vi "ROI entry-Event handler-Completion.vi"(11 "Ctrl ref of the control that caused the user event":refnum<vi>) -> (1 "Exit":bool=TRUE, 3 "Imaging Mode":T1)   [LabVIEW 2013]
uses:
  Typedefs/Top level VI states.ctl
  Visualisation/Functional Imaging Viewer/SubVIs/Experiment header interface/Typedefs/Header file type enum.ctl
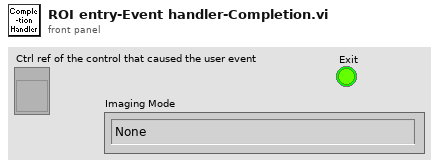
[diagram p1: front panel]
types:
  T1 = typedef "Top level VI states.ctl" = enum16{"None", "Initialise UI", "<STACK PROTOCOL STATES>", "AOL Zstack-START", "AOL Zstack-STOP", "Motor Zstack-START", "Motor Zstack-STOP", "<ACQUISITION PROTOCOL STATES> ", "Functional Acquisition-START", "Functional Acquisition-STOP", "Single Plane Acquisition-START", "Single Plane Acquisition-STOP", "Volume Acquisition-START", "Volume Acquisition-STOP", "<LIVE IMAGING PROTOCOL STATES>", "Live Imaging-START", "Live Imaging-STOP", "Live Plane Imaging-START", "Live Plane Imaging-STOP", "Live Volume Imaging-START", "Live Volume Imaging-STOP", "EXIT"}
  T2 = typedef "Header file type enum.ctl" = enum16{"All parameters", "Params for funct acq w ROI or mscn", "Params for funct acq w rectangles", "Live imaging header parameters", "AOL Parameters"}
  T3 = typedef "ROI parameters data type.ctl" = cluster{"ROI index":dbl, "ROI ID":dbl, "ROI Time (ns)":dbl, "Pixels in ROI":dbl, "X start":dbl, "Y start":dbl, "Z start":dbl, "X stop":dbl, "Y stop":dbl, "Z stop":dbl, "Angle (deg)":dbl, "Composite ID":dbl, "Number of lines":dbl, "Frame Size":dbl, "Zoom":dbl, "Laser Power (%)":dbl, "ROI group ID":dbl}
  T4 = typedef "AOL_Globals.ctl" = cluster{"Imaging Protocol":T5, "Number of POI":u16, "Number of Miniscans":u16, "Number of Trials":u16, "Number of Cycles ":u64, "# Averaged Frames":u16, "Laser power (%)":u8, "Pockels":dbl, "Acquisition Length (sec)":dbl, "Fill time (us)":dbl, "POI Dwell time (us)":dbl, "Miniscan Dwell time per pixel (us)":dbl, "PMT 1":dbl, "PMT 2":dbl, "Back Apperture":dbl, "Frame Size":T6, "Center Frequency":dbl, "Field of View":dbl, "DwellTime (us)":dbl, "Wavelength (nm)":dbl, "Zoom":dbl, "AOL Z":dbl, "AOL Mode":T7, "GridXY":dbl, "GridZ":dbl, "TriggerPeriod (sec)":dbl, "Number of Pixels in Miniscan":u16, "Experiment folder path":path, "X centre":dbl, "Y centre":dbl, "Angle (degrees)":dbl, "Plane Mode":T8, "Threshold":u16[], "Regenerate Chirps":bool, "Rectangle ROI length (pixels)":u16, "Rectangle ROI height (pixels)":u16, "AOD fill":u16, "Samples Wait after Trigger":u16, "StartUp Delay":i32, "Slip Cycle":u32, "Add Cycle":bool}
  T5 = typedef "Imaging Protocols enum.ctl" = enum16{"AOL Z-Stack", "Motor Z Stack", "Functional Acquisition", "Single Plane Acquisition", "Volume Acquisition", "Live Imaging", "Live Plane Imaging", "Live Volume Imaging"}
  T6 = typedef "Frame Size.ctl" = u16
  T7 = typedef "AOL modes.ctl" = enum16{"Raster", "Structural", "Pointing", "Mini Scan", "Alignment"}
  T8 = typedef "Plane Mode.ctl" = u16
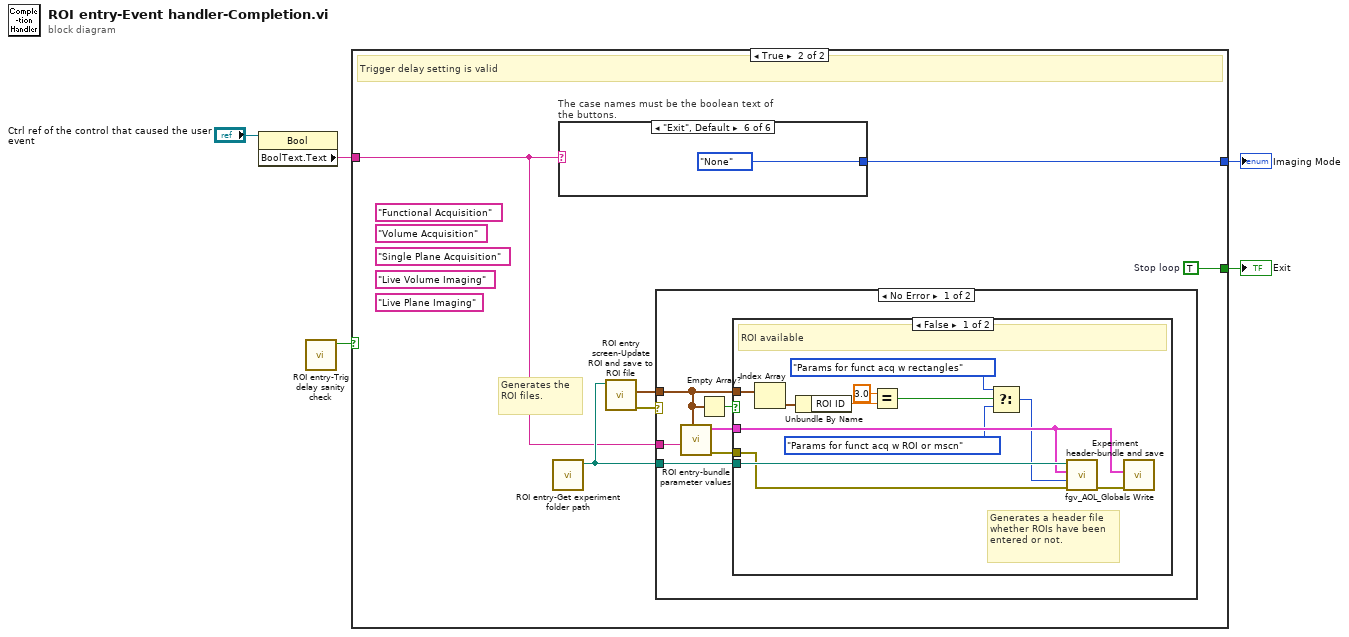
[diagram p0: block diagram]
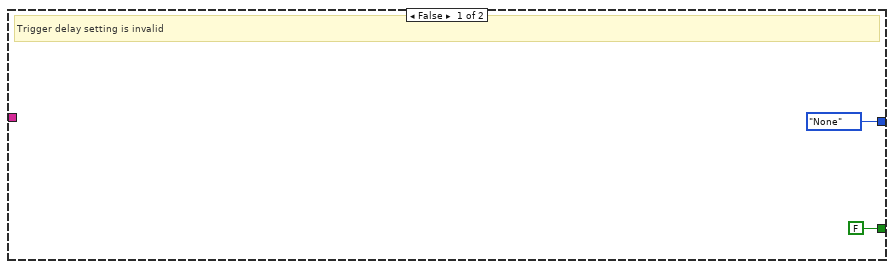
[diagram p2: hidden frame]
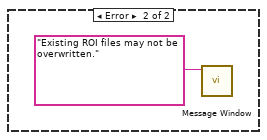
[diagram p4: hidden frame]
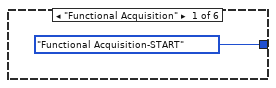
[diagram p5: hidden frame]
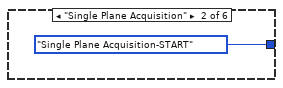
[diagram p6: hidden frame]
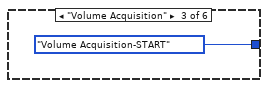
[diagram p7: hidden frame]
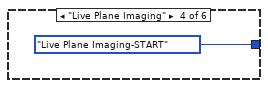
[diagram p8: hidden frame]
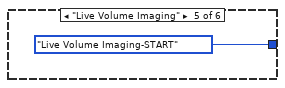
[diagram p9: hidden frame]
diagram:
  n1 = property on="Property Node" class="Bool"(reference="Ctrl ref of the control that caused the user event") -> ("BoolText.Text"=w5:string)  [unwired: 1 in, 2 out]
  n2 = call "ROI entry-Trig delay sanity check.vi"() -> ("Trigger delay is valid"=w1:bool)  [unwired: 10 in, 1 out]
  n3 = case shown="True" w1 {
    tunnel: w5 -> [_ w12]
    tunnel: [Top_level_VI_states."None" ("Imaging Mode") w9] -> w4
    tunnel: [FALSE ("Stop loop") w8] -> w2
    frame False {
      # "Trigger delay setting is invalid"
    }
    frame True {
      w8 = TRUE  # Stop loop
      (unwired) "Live Plane Imaging" ("Boolean Text.Text")
      (unwired) "Single Plane Acquisition" ("Boolean Text.Text")
      (unwired) "Live Volume Imaging" ("Boolean Text.Text")
      (unwired) "Functional Acquisition" ("Boolean Text.Text")
      (unwired) "Volume Acquisition" ("Boolean Text.Text")
      # "Generates the ROI files."
      # "Trigger delay setting is valid"
      n4 = call "ROI entry-Get experiment folder path.vi"() -> ("Experiment folder path"=w13:path)  [unwired: 10 in, 1 out]
      n5 = case "The case names must be the boolean text of the buttons." shown="\"Exit\", Default" w12 {
        tunnel: [Top_level_VI_states."Functional Acquisition-START" ("Imaging Mode") Top_level_VI_states."Single Plane Acquisition-START" ("Imaging Mode") Top_level_VI_states."Volume Acquisition-START" ("Imaging Mode") Top_level_VI_states."Live Plane Imaging-START" ("Imaging Mode") Top_level_VI_states."Live Volume Imaging-START" ("Imaging Mode") Top_level_VI_states."None" ("Imaging Mode")] -> w9
        frame "Functional Acquisition" {
        }
        frame "Single Plane Acquisition" {
        }
        frame "Volume Acquisition" {
        }
        frame "Live Plane Imaging" {
        }
        frame "Live Volume Imaging" {
        }
        frame "Exit", Default {
        }
      }
      n6 = call "ROI entry screen-Update ROI and save to ROI file.vi"("Experiment folder path"=w13) -> ("Error Out"=w11:errorcluster, "XYZ_Coordinates"=w10:T3[])  [unwired: 9 in]
      n7 = case shown="No Error" w11 {
        tunnel: w10 -> [w14 _]
        tunnel: w13 -> [w19 _]
        tunnel: w12 -> [w15 _]
        frame No Error {
          n8 = call "ROI entry-bundle parameter values.vi"("XYZ_Coordinates"=w14, "Button Label.Text"=w15) -> ("error out"=w17:errorcluster, "AOL_Globals out"=w18:T4)  [unwired: 8 in]
          n9 = Empty Array?(array=w14) -> (empty?=w16:bool)
          n10 = case shown="False" w16 {
            tunnel: w19 -> [w31 _]
            tunnel: w18 -> [w29 _]
            tunnel: w17 -> [w20 _]
            tunnel: w14 -> [w28 _]
            frame False {
              # "Generates a header file whether ROIs have been entered or not."
              # "ROI available"
              n11 = Index Array(array=w28) -> (element=w27:T3)  [unwired: 1 in]
              n12 = Unbundle By Name(w27) -> ("ROI ID"=w26:dbl)
              n13 = Equal?(x=3.0 ("y"), y=w26) -> (x = y?=w24:bool)
              n14 = Select(t=Header_file_type_enum."Params for funct acq w rectangles" ("Header file type"), s=w24, f=Header_file_type_enum."Params for funct acq w ROI or mscn" ("Header file type")) -> (s? t:f=w21:T2)
              n15 = call "Experiment header-bundle and save.vi"("error in (no error)"=w20, "Header file type"=w21, "AOL_Globals"=w29, "Experiment data folder path"=w31) -> ("error out"=w30:errorcluster)  [unwired: 7 in]
              n16 = call "fgv_AOL_Globals Write.vi"("error in (no error)"=w30, "AOL_Globals"=w29) -> ()  [unwired: 9 in, 1 out]
            }
            frame True {
              # "NO ROI ENTERED"
            }
          }
        }
        frame Error {
          n17 = call "Message Window.vi"("Message string"="Existing ROI files may not be overwritten.") -> ()  [unwired: 10 in, 1 out]
        }
      }
    }
  }
  "Imaging Mode" <- w4
  "Exit" <- w2
